vi "Jogging Speed.vi"(11 "String":string) -> (3 "F-format string":string)   [LabVIEW 2014, in "Programing Logic.lvclass"]
uses:
  Programing Logic.lvclass
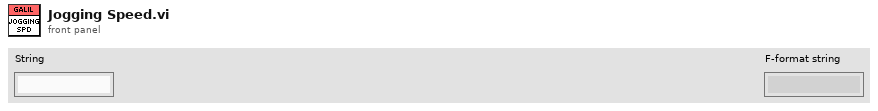
[diagram p1: front panel]
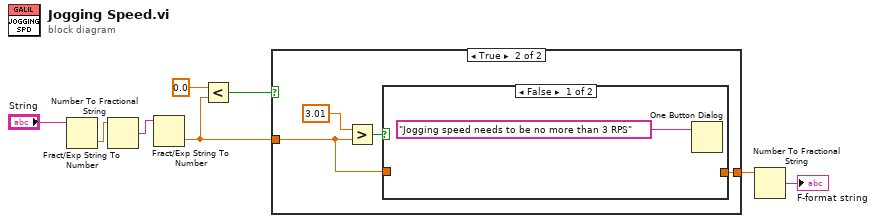
[diagram p0: block diagram]
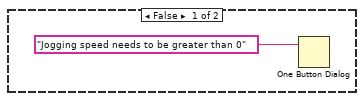
[diagram p2: hidden frame]
diagram:
  n1 = Fract/Exp String To Number(string="String") -> (number=w7:dbl)  [unwired: 3 in, 1 out]
  n2 = Number To Fractional String(number=w7) -> (F-format string=w2:string)  [unwired: 3 in]
  n3 = Fract/Exp String To Number(string=w2) -> (number=w4:dbl)  [unwired: 3 in, 1 out]
  n4 = Less?(x=0.0, y=w4) -> (x < y?=w5:bool)
  n5 = case shown="True" w5 {
    tunnel: w4 -> [_ w12]
    tunnel: [_ w11] -> w6
    frame False {
      n6 = One Button Dialog(message="Jogging speed needs to be greater than 0") -> ()  [unwired: 1 in, 1 out]
    }
    frame True {
      n7 = Greater?(x=3.01, y=w12) -> (0:w10:bool)
      n8 = case shown="False" w10 {
        tunnel: w12 -> [_ w15]
        tunnel: [_ w15] -> w11
        frame False {
          n9 = One Button Dialog(message="Jogging speed needs to be no more than 3 RPS") -> ()  [unwired: 1 in, 1 out]
        }
        frame True {
        }
      }
    }
  }
  n10 = Number To Fractional String(number=w6) -> (F-format string=→"F-format string":string)  [unwired: 3 in]
